vi "boolean2Index.vi"(11 "boolean":bool[](array[boolean])) -> (3 "index":i32[](array[numeric]))   [LabVIEW 2017]
panel:
  in  "Numeric":dbl
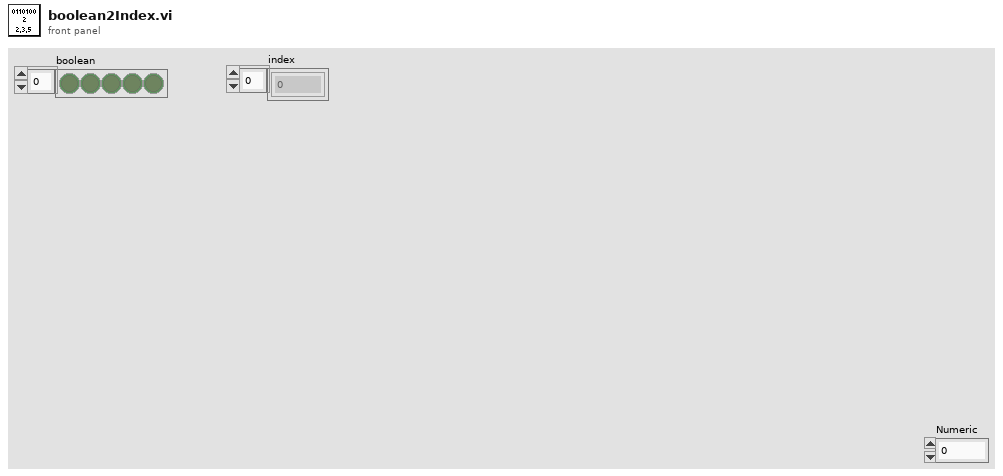
[diagram p1: front panel]
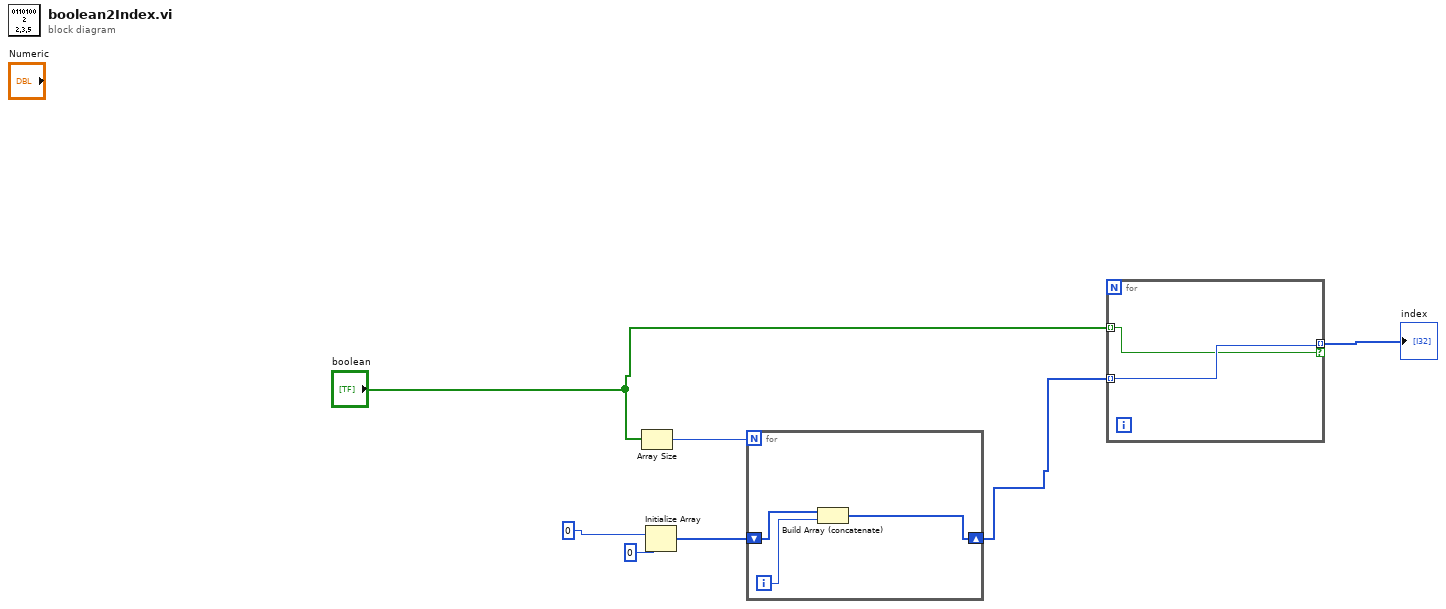
[diagram p0: block diagram]
diagram:
  n1 = Array Size(array="boolean") -> (size(s)=w7:i32)
  n2 = Initialize Array(0, 0 ("dimension size")) -> (w6:i32[])
  n3 = for {
    N: w7 -> [_]
    shift-right: [w9] -> w1
    shift-left: w6 -> [w10]
    i -> [w8]
    n4 = Build Array (concatenate)(w10, w8) -> (w9:i32[])
  }
  n5 = for {
    tunnel: w1 -> [w12] mode=indexing
    tunnel: "boolean" -> [w11] mode=indexing
    tunnel: [w12] -> w3 mode=indexing if=w11
  }
  "index" <- w3
